vi "Begin.vi"(11 "Image Size":T1=enum."160x120") -> (0 "error out":errorcluster)   [LabVIEW 2012]
doc: "Called before other user functions, this VI is expected to open initial I/O refnums, load in file data, and do all program initialization. Notice that the <B>error out</B> terminal is simply used for data flow. Wiring it to other structures or subVIs ensures that this VI runs first."
uses:
  <vilib>/Rock Robotics/WPI/Camera/WPI_CameraImageSize.ctl
  <vilib>/Rock Robotics/WPI/Camera/WPI_CameraWhite Balance Values.ctl
  <vilib>/Rock Robotics/WPI/Camera/WPI_CameraExposure Values.ctl
  <vilib>/Rock Robotics/WPI/Camera/WPI_CameraFrameRate.ctl
  <vilib>/Rock Robotics/WPI/DriverStation/WPI_DriverStationRobotMode2.ctl
  <vilib>/Rock Robotics/SystemInterfaces/DIO/FPGA_DIOPWMChannel.ctl
  <vilib>/Rock Robotics/WPI/Joystick/WPI_JoystickDeviceEnum.ctl
  <vilib>/Rock Robotics/SystemInterfaces/DIO/FPGA_DIOChannel.ctl
  <vilib>/Rock Robotics/SystemInterfaces/AI/FPGA_AIGyroChannel.ctl
  Robot Global Data.vi
  <vilib>/Rock Robotics/WPI/MotorControl/WPI_MotorControlOpen Victor.vi
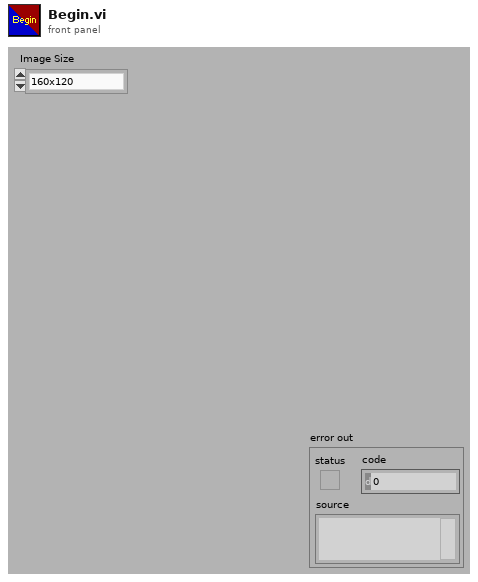
[diagram p1: front panel]
types:
  T1 = typedef "WPI_CameraImageSize.ctl" = enum16{"640x480", "320x240", "160x120"}
  T2 = typedef "FPGA_AIGyroChannel.ctl" = enum8{"AI 1", "AI 2", "Invalid"}
  T3 = typedef "FPGA_DIOChannel.ctl" = enum8{"DIO 1", "DIO 2", "DIO 3", "DIO 4", "DIO 5", "DIO 6", "DIO 7", "DIO 8", "DIO 9", "DIO 10", "DIO 11", "DIO 12", "DIO 13", "DIO 14", "Invalid"}
  T4 = typedef "WPI_JoystickDeviceEnum.ctl" = enum16{"USB 1", "USB 2", "USB 3", "USB 4", "Kinect 1", "Kinect 2"}
  T5 = typedef "FPGA_DIOPWMChannel.ctl" = enum8{"PWM 1", "PWM 2", "PWM 3", "PWM 4", "PWM 5", "PWM 6", "PWM 7", "PWM 8", "PWM 9", "PWM 10", "Invalid"}
  T6 = typedef "WPI_DriverStationRobotMode2.ctl" = enum16{"Autonomous Disabled", "Autonomous Enabled", "Teleop Disabled", "Teleop Enabled", "Timeout", "Finish", "Test Disabled", "Test Enabled"}
  T7 = typedef "WPI_CameraFrameRate.ctl" = u32
  T8 = typedef "WPI_CameraExposure Values.ctl" = enum16{"Auto", "Flicker-free 50 Hz", "Flicker-free 60 Hz", "Hold current"}
  T9 = typedef "WPI_CameraWhite Balance Values.ctl" = enum16{"Auto", "Fixed indoor", "Fixed outdoor 1", "Fixed outdoor 2", "Fixed fluorescent 1", "Fixed fluorescent 2", "Hold current"}
  T10 = typedef "WPI_CameraDevRef.ctl" = cluster{"Camera Address":string, "CameraStatus":errorcluster, "Acquire Image Notifier":refnum<notifier>}
  T11 = typedef "WPI_MotorControlDeviceRef.ctl" = cluster{"DeviceStatus":errorcluster, "Type":enum16{"PWM", "CAN"}, "PWM":cluster{"Digital Module":T12, "PWM Channel":T5, "DeadBand":T13}, "CAN":cluster{"Device Number":u8, "Control Mode":T14, "Semaphore":T15, "Max Vout":dbl}, "Invert":bool, "TransformRef":T16, "InvTransformRef":T16}
  T12 = typedef "FPGA_TypedefDigitalModule.ctl" = enum16{"Digital Module 1", "Digital Module 2"}
  T13 = typedef "WPI_PWMDeadband.ctl" = cluster{"Name":string, "maxPositivePwm":i32, "minPositivePwm":i32, "centerPwm":i32, "maxNegativePwm":i32, "minNegativePwm":i32, "angularRange":u16}
  T14 = typedef "WPI_CANJaguar_ControlMode.ctl" = enum8{"Percent VBus", "Current", "Speed", "Position", "Voltage"}
  T15 = typedef "Semaphore RefNum" = refnum<k1>
  T16 = typedef "WPI_PWMTransform_ConPane.ctl" = refnum<vi>
  T17 = typedef "WPI_ServoDeviceRef.ctl" = cluster{"DeviceStatus":errorcluster, "Digital Module":T12, "PWM Channel":T5, "DeadBand":T13}
  T18 = typedef "WPI_JoystickDevRef.ctl" = cluster{"Device":T4}
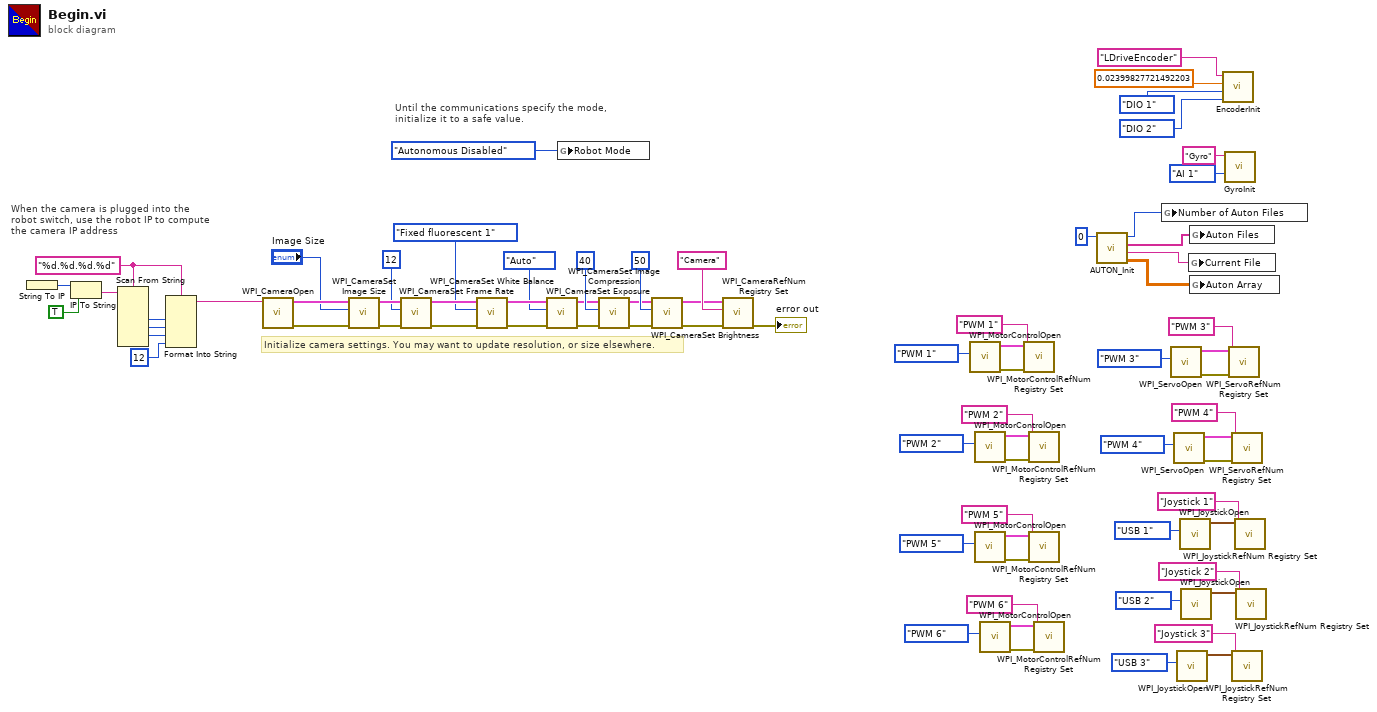
[diagram p0: block diagram]
diagram:
  w48 = "%d.%d.%d.%d" ("format string")
  # "Until the communications specify the mode,\ninitialize it to a safe value."
  # "When the camera is plugged into the\nrobot switch, use the robot IP to compute\nthe camera IP address"
  # "Initialize camera settings. You may want to update resolution, or size elsewhere."
  n1 = String To IP() -> (0:w55:u32)  [unwired: 1 in]
  n2 = IP To String(1:TRUE ("dot notation? (F)"), 2:w55) -> (0:w53:string)
  n3 = Scan From String(format string=w48, input string=w53) -> (output 1=w52:i32, output 2=w51:i32, output 3=w50:i32)  [unwired: 7 in, 3 out]
  n4 = Format Into String(format string=w48, w52, w51, w50, 12 ("Compression")) -> (resulting string=w46:string)  [unwired: 2 in, 1 out]
  n5 = call <vilib>:"WPI_CameraOpen.vi"("Camera Address"=w46) -> ("error out"=w67:errorcluster, "CameraDevRef"=w68:T10)  [unwired: 1 in, 8 out]
  n6 = call <vilib>:"WPI_CameraSet Image Size.vi"("error in (no error)"=w67, "Image Size"="Image Size", "CameraDevRef"=w68) -> ("error out"=w66:errorcluster, "CameraDevRef Out"=w69:T10)  [unwired: 7 out]
  n7 = call <vilib>:"WPI_CameraSet Frame Rate.vi"("error in (no error)"=w66, "Frame Rate (fps)"=T7 12, "CameraDevRef"=w69) -> ("error out"=w65:errorcluster, "CameraDevRef Out"=w71:T10)  [unwired: 7 out]
  n8 = call <vilib>:"WPI_CameraSet White Balance.vi"("error in (no error)"=w65, "White Balance"=WPI_CameraWhite_Balance_Values."Fixed fluorescent 1", "CameraDevRef"=w71) -> ("error out"=w64:errorcluster, "CameraDevRef Out"=w70:T10)  [unwired: 7 out]
  n9 = call <vilib>:"WPI_CameraSet Exposure.vi"("error in (no error)"=w64, "Exposure"=WPI_CameraExposure_Values."Auto", "CameraDevRef"=w70) -> ("error out"=w63:errorcluster, "CameraDevRef Out"=w73:T10)  [unwired: 7 out]
  n10 = global write "Robot Global Data.vi" "Robot Mode"(WPI_DriverStationRobotMode2."Autonomous Disabled" ("Robot Mode")) -> ()
  n11 = call <vilib>:"WPI_CameraSet Image Compression.vi"("error in (no error)"=w63, "Compression"=40, "CameraDevRef"=w73) -> ("error out"=w62:errorcluster, "CameraDevRef Out"=w72:T10)  [unwired: 7 out]
  n12 = call <vilib>:"WPI_CameraSet Brightness.vi"("error in (no error)"=w62, "Brightness"=50, "CameraDevRef"=w72) -> ("error out"=w60:errorcluster, "CameraDevRef Out"=w61:T10)  [unwired: 7 out]
  n13 = call <vilib>:"WPI_CameraRefNum Registry Set.vi"("error in (no error)"=w60, "refnum name"="Camera", "CameraDevRef"=w61) -> ("error out"=→"error out":errorcluster)  [unwired: 8 out]
  n14 = call-poly <vilib>:"WPI_MotorControlOpen.vi"("PWM Channel"=FPGA_DIOPWMChannel."PWM 1") -> ("error out"=w44:errorcluster, "MotorControlDeviceRef"=w43:T11)  [unwired: 9 in]
  n15 = call-poly <vilib>:"WPI_MotorControlOpen.vi"("PWM Channel"=FPGA_DIOPWMChannel."PWM 2") -> ("error out"=w37:errorcluster, "MotorControlDeviceRef"=w38:T11)  [unwired: 9 in]
  n16 = call-poly <vilib>:"WPI_MotorControlOpen.vi"("PWM Channel"=FPGA_DIOPWMChannel."PWM 5") -> ("error out"=w29:errorcluster, "MotorControlDeviceRef"=w30:T11)  [unwired: 9 in]
  n17 = call-poly <vilib>:"WPI_MotorControlOpen.vi"("PWM Channel"=FPGA_DIOPWMChannel."PWM 6") -> ("error out"=w36:errorcluster, "MotorControlDeviceRef"=w35:T11)  [unwired: 9 in]
  n18 = call <vilib>:"WPI_MotorControlRefNum Registry Set.vi"("error in (no error)"=w44, "refnum name"="PWM 1", "MotorControlDevRef"=w43) -> ()  [unwired: 7 in, 2 out]
  n19 = call <vilib>:"WPI_MotorControlRefNum Registry Set.vi"("error in (no error)"=w37, "refnum name"="PWM 2", "MotorControlDevRef"=w38) -> ()  [unwired: 7 in, 2 out]
  n20 = call <vilib>:"WPI_MotorControlRefNum Registry Set.vi"("error in (no error)"=w29, "refnum name"="PWM 5", "MotorControlDevRef"=w30) -> ()  [unwired: 7 in, 2 out]
  n21 = call <vilib>:"WPI_MotorControlRefNum Registry Set.vi"("error in (no error)"=w36, "refnum name"="PWM 6", "MotorControlDevRef"=w35) -> ()  [unwired: 7 in, 2 out]
  n22 = call "AUTON_Init.vi"("Default File"=0) -> ("Auton Array"=w7:dbl[][], "Current File"=w8:string, "Auton Files"=w9:string[], "Number of Auton Files"=w10:i64)  [unwired: 7 in]
  n23 = global write "Robot Global Data.vi" "Number of Auton Files"(w10) -> ()
  n24 = call <vilib>:"WPI_ServoOpen.vi"("PWM Channel"=FPGA_DIOPWMChannel."PWM 3") -> ("error out"=w28:errorcluster, "ServoDeviceRef"=w27:T17)  [unwired: 9 in]
  n25 = call <vilib>:"WPI_ServoOpen.vi"("PWM Channel"=FPGA_DIOPWMChannel."PWM 4") -> ("error out"=w21:errorcluster, "ServoDeviceRef"=w22:T17)  [unwired: 9 in]
  n26 = call <vilib>:"WPI_JoystickOpen.vi"("JoystickDevice"=WPI_JoystickDeviceEnum."USB 3") -> ("JoystickDevRef"=w14:T18)  [unwired: 10 in]
  n27 = call <vilib>:"WPI_JoystickOpen.vi"("JoystickDevice"=WPI_JoystickDeviceEnum."USB 1") -> ("JoystickDevRef"=w20:T18)  [unwired: 10 in]
  n28 = call <vilib>:"WPI_JoystickOpen.vi"("JoystickDevice"=WPI_JoystickDeviceEnum."USB 2") -> ("JoystickDevRef"=w15:T18)  [unwired: 10 in]
  n29 = global write "Robot Global Data.vi" "Current File"(w8) -> ()
  n30 = global write "Robot Global Data.vi" "Auton Files"(w9) -> ()
  n31 = global write "Robot Global Data.vi" "Auton Array"(w7) -> ()
  n32 = call "EncoderInit.vi"("refnum name"="LDriveEncoder", "DistancePerCount"=0.02399827721492203, "DIO Channel"=FPGA_DIOChannel."DIO 1", "DIO Channel 2"=FPGA_DIOChannel."DIO 2") -> ()  [unwired: 7 in]
  n33 = call "GyroInit.vi"("refnum name"="Gyro", "Analog Channel"=FPGA_AIGyroChannel."AI 1") -> ()  [unwired: 8 in]
  n34 = call <vilib>:"WPI_ServoRefNum Registry Set.vi"("error in (no error)"=w28, "refnum name"="PWM 3", "ServoDeviceRef"=w27) -> ()  [unwired: 7 in, 2 out]
  n35 = call <vilib>:"WPI_ServoRefNum Registry Set.vi"("error in (no error)"=w21, "refnum name"="PWM 4", "ServoDeviceRef"=w22) -> ()  [unwired: 7 in, 2 out]
  n36 = call <vilib>:"WPI_JoystickRefNum Registry Set.vi"("refnum name"="Joystick 3", "JoystickDevRef"=w14) -> ()  [unwired: 8 in, 2 out]
  n37 = call <vilib>:"WPI_JoystickRefNum Registry Set.vi"("refnum name"="Joystick 1", "JoystickDevRef"=w20) -> ()  [unwired: 8 in, 2 out]
  n38 = call <vilib>:"WPI_JoystickRefNum Registry Set.vi"("refnum name"="Joystick 2", "JoystickDevRef"=w15) -> ()  [unwired: 8 in, 2 out]
